vi "Set Output State.vi"(8 "error in (no error)":errorcluster, 10 "Output State":bool, 11 "Cooler in":refnum<class "Cooler.lvclass">) -> (0 "error out":errorcluster, 3 "Cooler out":refnum<class "Cooler.lvclass">)   [LabVIEW 2012, in "Cooler.lvlib" / "Cooler.lvclass"]
uses:
  Cooler.lvclass
  Simulation/Simulation Data_Global.vi
  Simulation/Simulation.lvlib
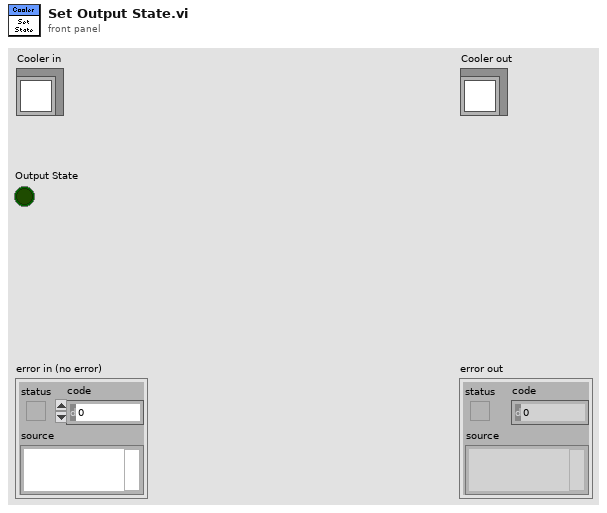
[diagram p1: front panel]
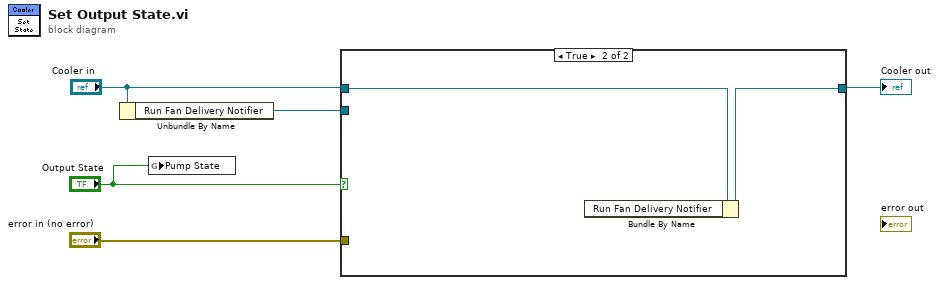
[diagram p0: block diagram]
diagram:
  n1 = Unbundle By Name("Cooler in") -> ("Run Fan Delivery Notifier"=w3:refnum<notifier>)
  n2 = global write "Simulation Data_Global.vi" "Pump State"("Output State") -> ()
  n3 = case shown="True" "Output State" {
    tunnel: "error in (no error)" -> [w7 _]
    tunnel: "Cooler in" -> [w9 w12]
    tunnel: [w9 w11] -> w4
    tunnel: w3 -> [w6 _]
    frame False {
      n4 = flat-sequence {
        tunnel: w6 -> [_]
        tunnel: [w10] -> w8
        tunnel: w7 -> [w10]
        tunnel: w8 -> [_]
        frame #0 {
        }
        frame #1 {
        }
      }
    }
    frame True {
      n5 = Bundle By Name(cluster=w12) -> (w11:refnum<class "Cooler.lvclass">)  [unwired: 1 in]
    }
  }
  "Cooler out" <- w4
